vi "Set TWM Processing.vi"(4 "status ref (none)":refnum<vi>, 7 "TWM Measurement properties":T1={"Sampling frequency (Hz)"=500000.0, "Record length (multiples of period)"=1000.0, "Signal amplitude (V)"=4.5, "Measurement frequency (Hz)"=1000.0, "Calculate RMS from samples"=FALSE, "Algorithm"="TWM-WFFT", "Measurement path"=""} {"Measurement frequency (Hz)" format="%#_3p"; "Record length (multiples of period)" format="%#_3p"; "Sampling frequency (Hz)" format="%#_3p"}, 8 "error in":errorcluster, 11 "handle":i32) -> (0 "error out":errorcluster, 3 "handle out":i32)   [LabVIEW 2020]
doc: "Sets data processing in TWM. Sets algorithm and parameters."
uses:
  external libraries/TWM-1.8.7.0-client/TWM Client Meas Setup.ctl
  external libraries/TWM-1.8.7.0-client/TWM Client Meas Setup Trig.ctl
  external libraries/TWM-1.8.7.0-client/TWM Client Processing Setup.ctl
  external libraries/TWM-1.8.7.0-client/TWM Client.lvlib
  Type definitions/Sampling properties.ctl
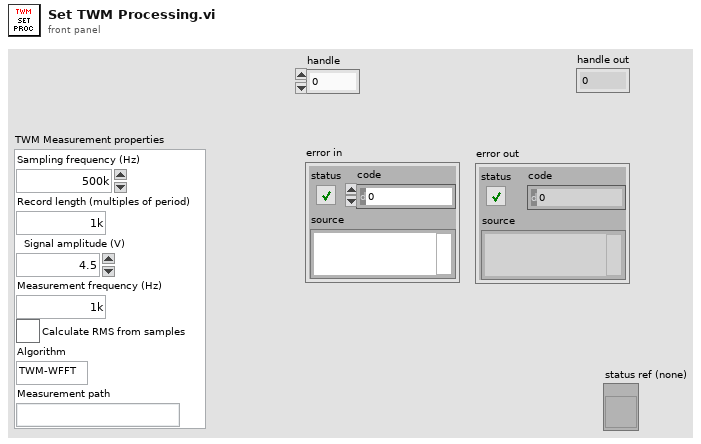
[diagram p1: front panel]
types:
  T1 = typedef "Sampling properties.ctl" = cluster{"Sampling frequency (Hz)":dbl, "Record length (multiples of period)":dbl, "Signal amplitude (V)":dbl, "Measurement frequency (Hz)":dbl, "Calculate RMS from samples":bool, "Algorithm":string, "Measurement path":string}
  T2 = typedef "TWM Client.lvlib/TWM Client Processing Setup.ctl" = cluster{"calculate":i32, "all cycles at once":bool, "alg. ID":string, "unc mode":string, "mc cycles":i32, "timeout [s]":dbl, "loc [-]":dbl, "valid?":bool, "qwtb params":cluster{"name":string, "data":string[]}[]}
  T3 = typedef "TWM Client.lvlib/TWM Client Meas Setup Trig.ctl" = cluster{"valid?":bool, "coupling (T is DC)":bool, "slope (T is positive)":bool, "source (Immediate)":enum16{"Immediate", "Level", "External"}, "level [V]":dbl, "hysteresis [V]":dbl, "pre-trigger [%]":dbl}
  T4 = typedef "TWM Client.lvlib/TWM Client Meas Setup.ctl" = cluster{"smpl count":i32, "smpl rate [Hz]":dbl, "average":i32, "aperture [s]":dbl, "valid?":bool, "meas fld":path, "sub-records":i32, "ranges [Vpk]":dbl[], "smpl rate - fr [Hz]":dbl, "smpl rate - div":dbl, "smpl rate - mul":dbl, "offsets [V]":dbl[]}
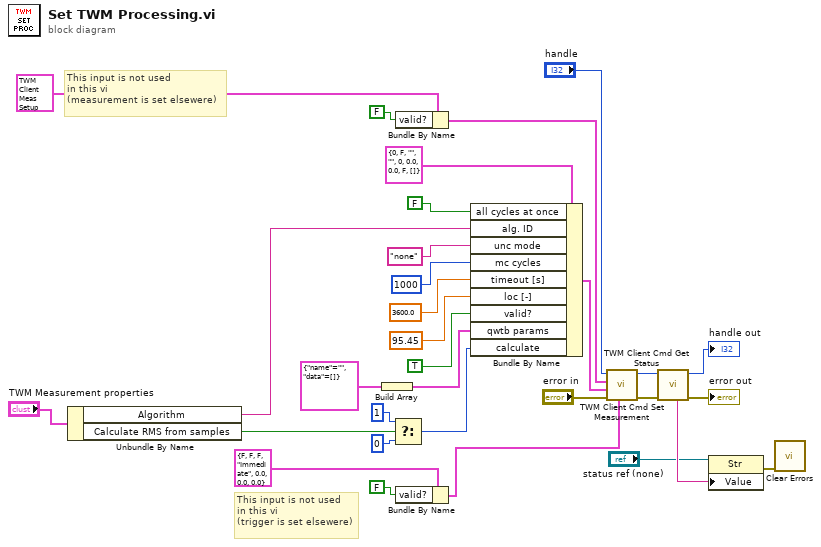
[diagram p0: block diagram]
diagram:
  # "This input is not used\nin this vi\n(trigger is set elsewere)"
  # "This input is not used\nin this vi\n(measurement is set elsewere)"
  n1 = Unbundle By Name("TWM Measurement properties") -> ("Algorithm"=w1:string, "Calculate RMS from samples"=w2:bool)
  n2 = Build Array(cluster{"name":string, "data":string[]} {"name"="", "data"=[]} ("Cluster")) -> (w4:cluster{"name":string, "data":string[]}[])
  n3 = Select(t=1 ("calculate"), s=w2, f=0 ("calculate")) -> (s? t:f=w8:i32)
  n4 = Bundle By Name(cluster=T4 {"smpl count"=0, "smpl rate [Hz]"=0.0, "average"=0, "aperture [s]"=0.0, "valid?"=FALSE, "meas fld"=path "", "sub-records"=0, "ranges [Vpk]"=[], "smpl rate - fr [Hz]"=0.0, "smpl rate - div"=0.0, "smpl rate - mul"=0.0, "offsets [V]"=[]} ("meas"), "valid?"=FALSE) -> (w29:T4)
  n5 = Bundle By Name(cluster=T3 {"valid?"=FALSE, "coupling (T is DC)"=FALSE, "slope (T is positive)"=FALSE, "source (Immediate)"=enum."Immediate", "level [V]"=0.0, "hysteresis [V]"=0.0, "pre-trigger [%]"=0.0} ("Trigger"), "valid?"=FALSE) -> (w27:T3)
  n6 = Bundle By Name(cluster=T2 {"calculate"=0, "all cycles at once"=FALSE, "alg. ID"="", "unc mode"="", "mc cycles"=0, "timeout [s]"=0.0, "loc [-]"=0.0, "valid?"=FALSE, "qwtb params"=[]} ("processing"), "all cycles at once"=FALSE, "alg. ID"=w1, "unc mode"="none", "mc cycles"=1000, "timeout [s]"=3600.0, "loc [-]"=95.45, "valid?"=TRUE, "qwtb params"=w4, "calculate"=w8) -> (w24:T2)
  n7 = call "TWM Client Cmd Set Measurement.vi"("Trigger"=w27, "error in"="error in", "processing"=w24, "meas"=w29, "handle"="handle") -> ("error out"=w15:errorcluster, "handle out"=w14:i32)  [unwired: 5 in]
  n8 = call "TWM Client Cmd Get Status.vi"("error in"=w15, "handle"=w14) -> ("error out"=→"error out":errorcluster, "handle out"=→"handle out":i32, "status string"=w11:string)  [unwired: 5 in, 2 out]
  n9 = property class="Str"(reference="status ref (none)", "Value"=w11) -> (error out=w16:errorcluster)  [unwired: 1 in, 1 out]
  n10 = call <vilib>:"Clear Errors.vi"("error in (no error)"=w16) -> ()  [unwired: 5 in, 2 out]
